vi "温度补偿.vi"() -> ()   [LabVIEW 2016, in "斯坦道CODMn.lvlib"]
uses:
  <vilib>/Analysis/6fits.llb/Curve Fitting Criteria.ctl
  <vilib>/Plasmionique/MB Master/MB Master.lvlib
  <vilib>/Analysis/NI_AALPro.lvlib
panel:
  in  "读取":bool
  in  "写入":bool
  in  "关闭":bool
  in  "曲线模型":T1 {"二次方程"."x^2" format="%#.6g"; "二次方程"."K" format="%#.6g"; "二次方程"."B" format="%#.6g"; "r^2" format="%.7f"; "测量吸光度5" format="%#.6f"; "测量吸光度4" format="%#.6f"; "测量吸光度3" format="%#.6f"; "测量吸光度2" format="%#.6f"; "测量吸光度1" format="%#.6f"}
  # "温度"
  # "滴定数"
  # "温度一"
  # "温度二"
  # "温度三"
  # "温度四"
  # "温度五"
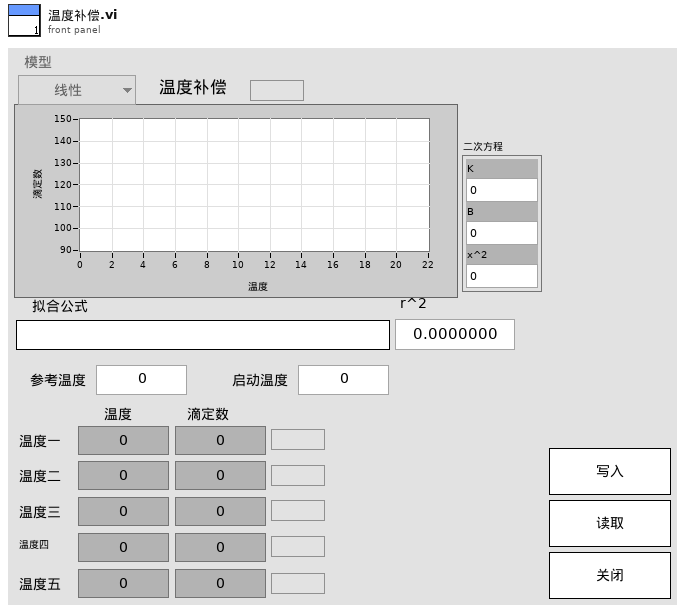
[diagram p1: front panel]
types:
  T1 = cluster{"标液浓度1":dbl, "测量吸光度1":dbl, "样品1启用":bool, "标液浓度2":dbl, "测量吸光度2":dbl, "样品2启用":bool, "标液浓度3":dbl, "测量吸光度3":dbl, "样品3启用":bool, "标液浓度4":dbl, "测量吸光度4":dbl, "样品4启用":bool, "标液浓度5":dbl, "测量吸光度5":dbl, "样品5启用":bool, "模型":enum32{"线性", "多项式", "折线"}, "XY图":cluster{"X Values":dbl[], "Y Values":dbl[]}[], "拟合公式":string, "r^2":dbl, "二次方程":cluster{"K":dbl, "B":dbl, "x^2":dbl}, "参考温度":dbl, "温度补偿":bool, "启动温度":dbl}
  T2 = typedef "NI_AALPro.lvlib/Curve Fitting Criteria.ctl" = u16
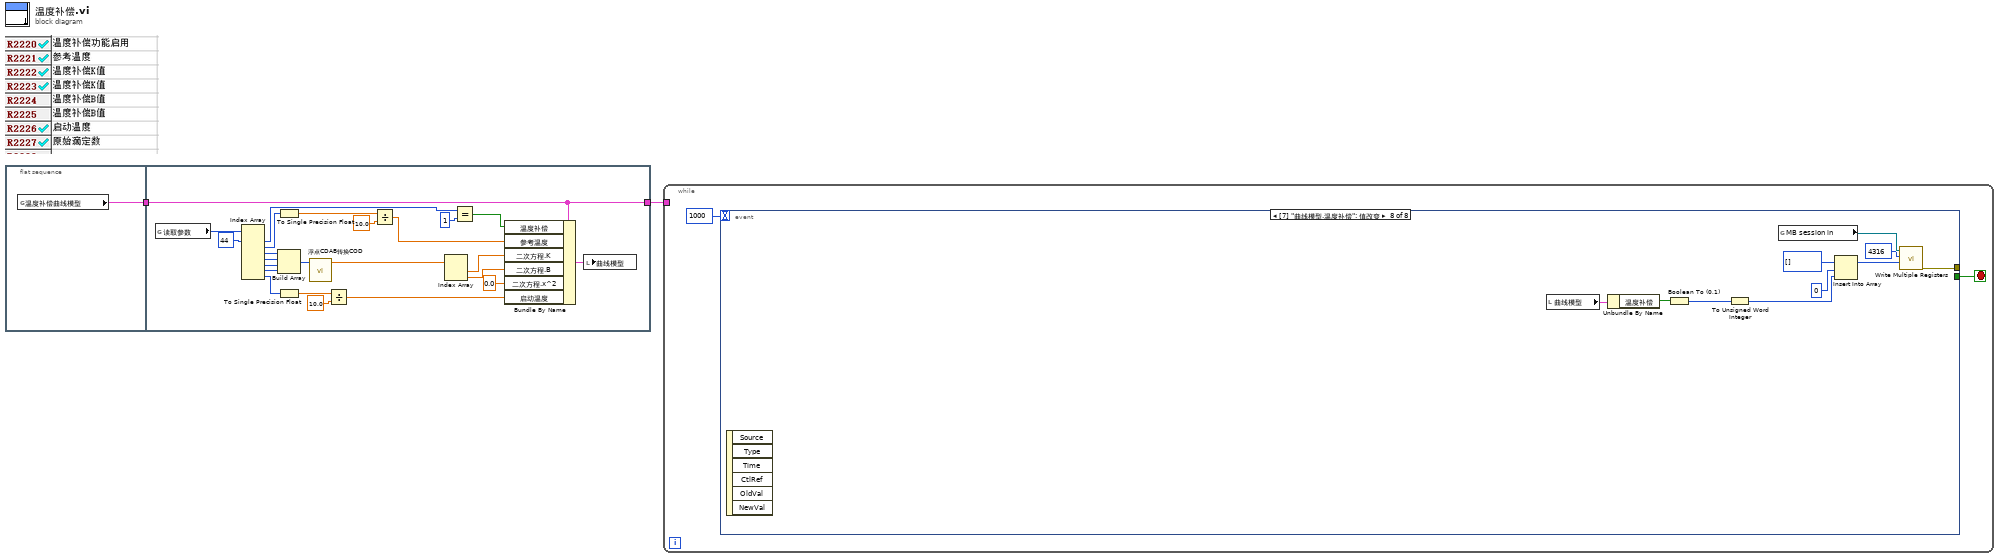
[diagram p0: block diagram]
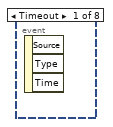
[diagram p2: hidden frame]
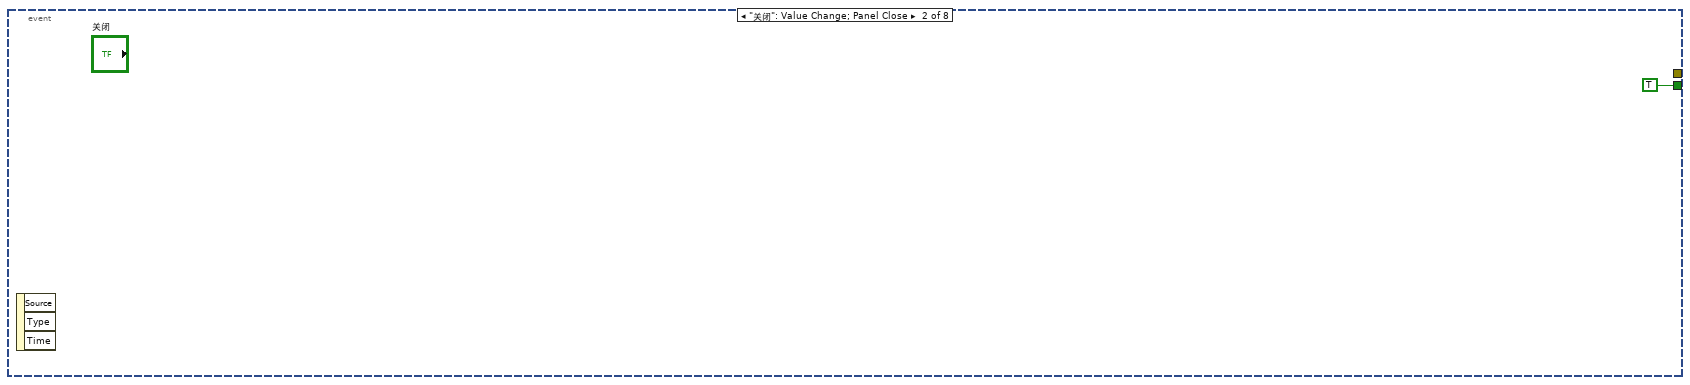
[diagram p3: hidden frame]
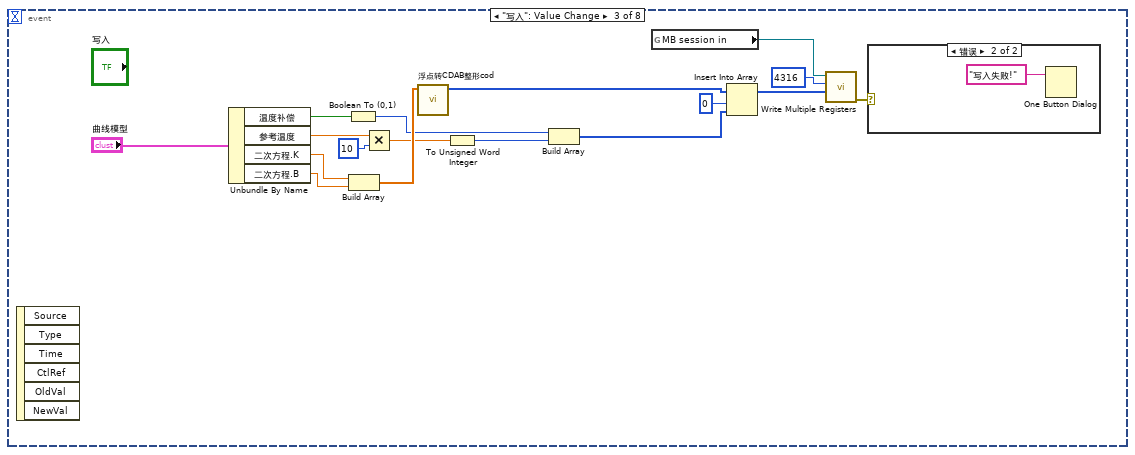
[diagram p4: hidden frame]
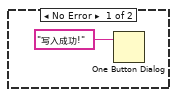
[diagram p5: hidden frame]
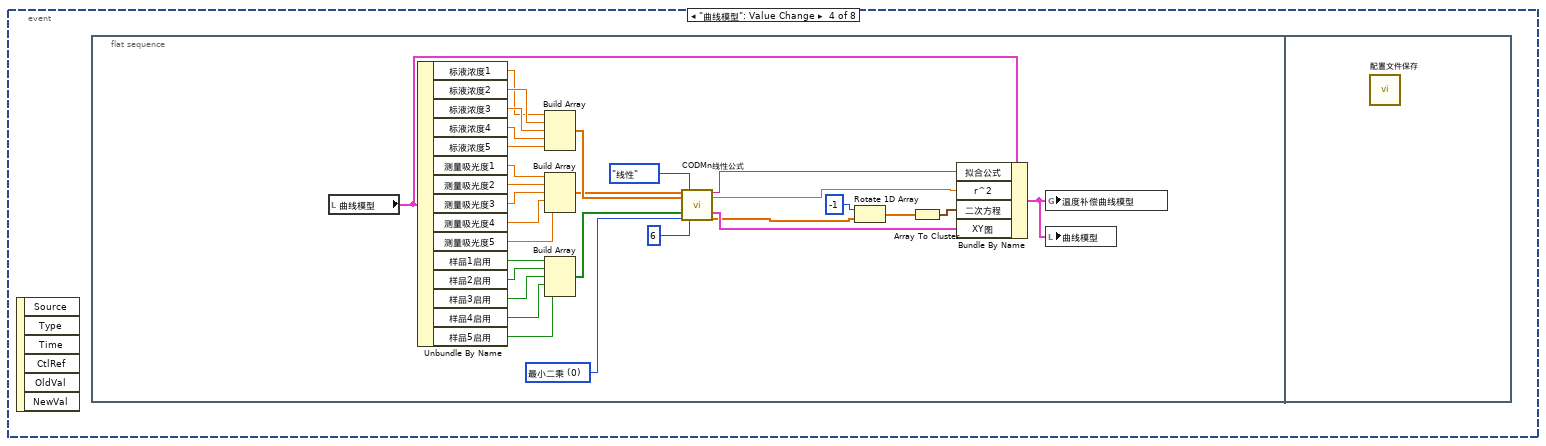
[diagram p6: hidden frame]
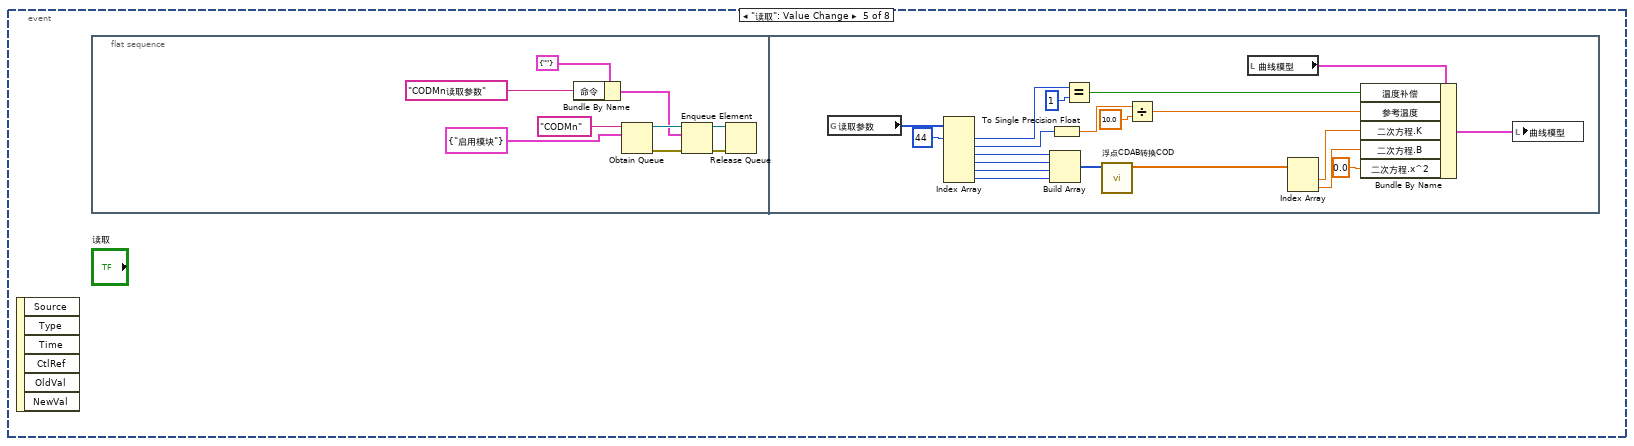
[diagram p7: hidden frame]
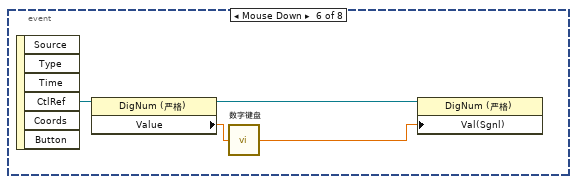
[diagram p8: hidden frame]
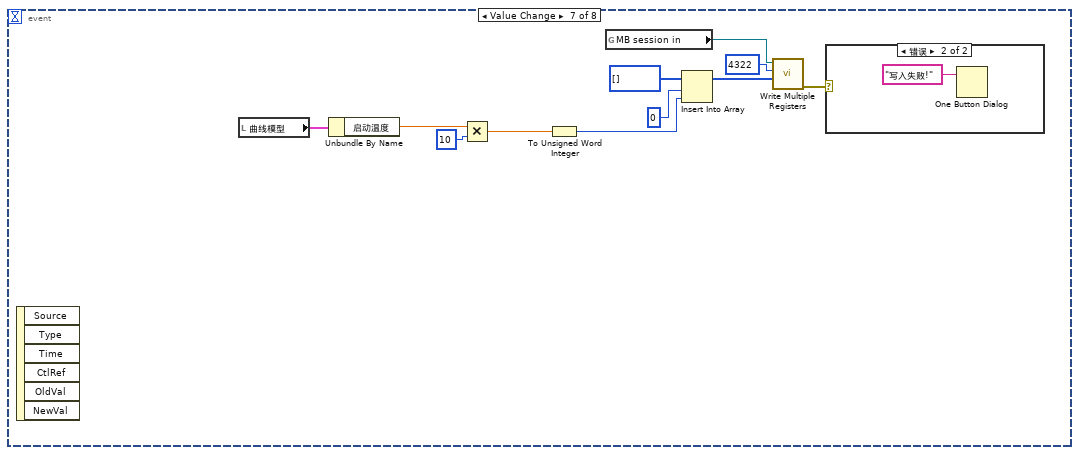
[diagram p9: hidden frame]
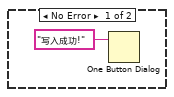
[diagram p10: hidden frame]
diagram:
  n1 = flat-sequence {
    tunnel: [w3] -> w1
    tunnel: [w25] -> w2
    tunnel: w1 -> [w25]
    frame #0 {
      n2 = global read "CODMn断电保存全局变量.vi" "温度补偿曲线模型"() -> (w3:T1)
    }
    frame #1 {
      n3 = global read "COD内部交互全局.vi" "读取参数"() -> (w27:u16[])
      n4 = Index Array(array=w27, index #1=44 ("索引")) -> (element #1=w12:u16, element #2=w9:u16, element #3=w22:u16, element #4=w21:u16, element #5=w20:u16, element #6=w19:u16, element #7=w5:u16)  [unwired: 6 in]
      n5 = To Single Precision Float(number=w9) -> (single precision float=w8:sgl)
      n6 = Build Array(w22, w21, w20, w19) -> (w18:u16[])
      n7 = To Single Precision Float(number=w5) -> (single precision float=w7:sgl)
      n8 = call "浮点CDAB转换COD.vi"("数组"=w18) -> ("数组 2"=w17:sgl[])  [unwired: 10 in]
      n9 = Divide(x=w7, y=sgl 10.0) -> (x/y=w4:sgl)
      n10 = Divide(x=w8, y=sgl 10.0) -> (x/y=w23:sgl)
      n11 = Index Array(array=w17) -> (element #1=w16:sgl, element #2=w15:sgl)  [unwired: 2 in]
      n12 = Equal?(x=w12, y=u16 1) -> (x = y?=w10:bool)
      n13 = Bundle By Name(cluster=w25, "温度补偿"=w10, "参考温度"=w23, "二次方程.K"=w16, "二次方程.B"=w15, "二次方程.x^2"=0.0, "启动温度"=w4) -> (w24:T1)
      n14 = local write "曲线模型"(w24) -> ()
    }
  }
  n15 = while {
    tunnel: w2 -> [_]
    stop <- w29 stop-if-true
    n16 = event shown="[7] \"曲线模型.温度补偿\": 值改变" {
      selector: _ -> [_ _ _ _ _ _ _ _]
      dyn-events: _ -> [_ _ _ _ _ _ _ _]
      timeout: 1000 -> [_ _ _ _ _ _ _ _]
      tunnel: [_ TRUE _ _ _ _ _ _] -> w29
      tunnel: [_ _ _ _ _ _ _ w126] -> _
      event Timeout {
        n17 = event-data() -> ()  [unwired: 1 in, 3 out]
      }
      event "关闭": Value Change; Panel Close {
        n18 = event-data() -> ()  [unwired: 1 in, 3 out]
      }
      event "写入": Value Change {
        n19 = event-data() -> ()  [unwired: 1 in, 6 out]
        n20 = Unbundle By Name("曲线模型") -> ("温度补偿"=w34:bool, "参考温度"=w40:dbl, "二次方程.K"=w44:dbl, "二次方程.B"=w43:dbl)
        n21 = Boolean To (0,1)(Boolean=w34) -> (0, 1=w33:i16)
        n22 = Build Array(w44, w43) -> (w42:dbl[])
        n23 = Multiply(x=w40, y=u16 10 ("新元素/子数组")) -> (x*y=w38:dbl)
        n24 = call "浮点转CDAB整形cod.vi"("浮点数"=w42) -> ("CDAB整形输出"=w31:u16[])  [unwired: 10 in]
        n25 = To Unsigned Word Integer(number=w38) -> (unsigned 16bit integer=w35:u16)
        n26 = Build Array(w33, w35) -> (w32:u16[])
        n27 = global read "COD浓度全局变量.vi" "MB session in"() -> (w46:refnum<class "MB_Master.lvclass">)
        n28 = Insert Into Array(array=w31, index=0 ("索引"), new element=w32) -> (w37:u16[])
        n29 = call <vilib>:"Write Multiple Registers.vi"("values"=w37, "starting address"=u16 4316, "MB session in"=w46) -> ("error out"=w36:errorcluster)  [unwired: 7 in, 1 out]
        n30 = case shown="错误" w36 {
          frame No Error {
            n31 = One Button Dialog(message="写入成功!" ("消息")) -> ()  [unwired: 1 in, 1 out]
          }
          frame Error {
            n32 = One Button Dialog(message="写入失败!" ("消息")) -> ()  [unwired: 1 in, 1 out]
          }
        }
      }
      event "曲线模型": Value Change {
        n33 = event-data() -> ()  [unwired: 1 in, 6 out]
        n34 = flat-sequence {
          frame #0 {
            w51 = T2 0 items=["最小二乘", "最小绝对残差", "Bisquare"] ("method")
            n35 = local read "曲线模型"() -> (w72:T1)
            n36 = Unbundle By Name(w72) -> ("标液浓度1"=w54:dbl, "标液浓度2"=w55:dbl, "标液浓度3"=w56:dbl, "标液浓度4"=w57:dbl, "标液浓度5"=w58:dbl, "测量吸光度1"=w59:dbl, "测量吸光度2"=w60:dbl, "测量吸光度3"=w61:dbl, "测量吸光度4"=w62:dbl, "测量吸光度5"=w63:dbl, "样品1启用"=w64:bool, "样品2启用"=w65:bool, "样品3启用"=w66:bool, "样品4启用"=w67:bool, "样品5启用"=w68:bool)
            n37 = Build Array(w54, w55, w56, w57, w58) -> (w71:dbl[])
            n38 = Build Array(w59, w60, w61, w62, w63) -> (w70:dbl[])
            n39 = Build Array(w64, w65, w66, w67, w68) -> (w69:bool[])
            n40 = call "CODMn线性公式.vi"("标液浓度"=w70, "滴定数"=w71, "启用"=w69, "method"=w51, "模型"=enum32{"线性", "多项式", "折线"}."线性", "精度"=6) -> ("拟合方程"=w73:string, "r^2"=w74:dbl, "XY图"=w79:cluster{"X Values":dbl[], "Y Values":dbl[]}[], "Polynomial Coefficients"=w78:dbl[])  [unwired: 7 in, 3 out]
            n41 = Rotate 1D Array(1:w78, 2:-1 ("n")) -> (0:w75:dbl[])
            n42 = Array To Cluster(array=w75) -> (cluster=w77:cluster{"[0]":dbl, "[1]":dbl, "[2]":dbl})
            n43 = Bundle By Name(cluster=w72, "拟合公式"=w73, "r^2"=w74, "二次方程"=w77, "XY图"=w79) -> (w50:T1)
            n44 = global write "CODMn断电保存全局变量.vi" "温度补偿曲线模型"(w50) -> ()
            n45 = local write "曲线模型"(w50) -> ()
          }
          frame #1 {
            n46 = call "配置文件保存.vi"() -> ()  [unwired: 12 in]
          }
        }
      }
      event "读取": Value Change {
        n47 = event-data() -> ()  [unwired: 1 in, 6 out]
        n48 = flat-sequence {
          frame #0 {
            n49 = Bundle By Name(cluster=cluster{"命令":string} {"命令"=""} ("元素"), "命令"="CODMn读取参数" ("名称（未命名）")) -> (w82:cluster{"命令":string})
            n50 = Obtain Queue(name (unnamed)="CODMn", element data type=cluster{"命令":string} {"命令"="启用模块"} ("元素")) -> (queue out=w87:refnum<queue>, error out=w88:errorcluster)  [unwired: 3 in, 1 out]
            n51 = Enqueue Element(queue=w87, element=w82, error in (no error)=w88) -> (queue out=w85:refnum<queue>, error out=w86:errorcluster)  [unwired: 1 in, 1 out]
            n52 = Release Queue(queue=w85, error in (no error)=w86) -> ()  [unwired: 1 in, 3 out]
          }
          frame #1 {
            n53 = global read "COD内部交互全局.vi" "读取参数"() -> (w92:u16[])
            n54 = Index Array(array=w92, index #1=44 ("索引")) -> (element #1=w106:u16, element #2=w90:u16, element #3=w96:u16, element #4=w97:u16, element #5=w98:u16, element #6=w99:u16)  [unwired: 5 in]
            n55 = Build Array(w96, w97, w98, w99) -> (w100:u16[])
            n56 = To Single Precision Float(number=w90) -> (single precision float=w89:sgl)
            n57 = Equal?(x=w106, y=u16 1) -> (x = y?=w108:bool)
            n58 = call "浮点CDAB转换COD.vi"("数组"=w100) -> ("数组 2"=w101:sgl[])  [unwired: 10 in]
            n59 = Divide(x=w89, y=sgl 10.0) -> (x/y=w95:sgl)
            n60 = local read "曲线模型"() -> (w91:T1)
            n61 = Index Array(array=w101) -> (element #1=w102:sgl, element #2=w103:sgl)  [unwired: 2 in]
            n62 = Bundle By Name(cluster=w91, "温度补偿"=w108, "参考温度"=w95, "二次方程.K"=w102, "二次方程.B"=w103, "二次方程.x^2"=0.0) -> (w94:T1)
            n63 = local write "曲线模型"(w94) -> ()
          }
        }
      }
      event "曲线模型.标液浓度1", "曲线模型.测量吸光度1", "曲线模型.标液浓度2", "曲线模型.测量吸光度2", "曲线模型.标液浓度3", "曲线模型.测量吸光度3", "曲线模型.标液浓度4", "曲线模型.测量吸光度4", "曲线模型.标液浓度5", "曲线模型.测量吸光度5", "曲线模型.参考温度", "曲线模型.启动温度": Mouse Down {
        n64 = event-data() -> ("CtlRef"=w112:refnum<vi>)  [unwired: 1 in, 5 out]
        n65 = property class="DigNum (严格)"(reference=w112) -> (reference out=w110:refnum<vi>, "Value"=w111:dbl)  [unwired: 1 in, 1 out]
        n66 = call "数字键盘.vi"("OldNumber"=w111) -> ("NewNumber"=w109:sgl)
        n67 = property class="DigNum (严格)"(reference=w110, "Val(Sgnl)"=w109) -> ()  [unwired: 1 in, 2 out]
      }
      event "曲线模型.启动温度": Value Change {
        n68 = event-data() -> ()  [unwired: 1 in, 6 out]
        n69 = local read "曲线模型"() -> (w123:T1)
        n70 = Unbundle By Name(w123) -> ("启动温度"=w115:dbl)
        n71 = Multiply(x=w115, y=u16 10 ("新元素/子数组")) -> (x*y=w116:dbl)
        n72 = To Unsigned Word Integer(number=w116) -> (unsigned 16bit integer=w114:u16)
        n73 = global read "COD浓度全局变量.vi" "MB session in"() -> (w122:refnum<class "MB_Master.lvclass">)
        n74 = Insert Into Array(array=u16[] [] ("CDAB整形输出"), index=0 ("索引"), new element=w114) -> (w119:u16[])
        n75 = call <vilib>:"Write Multiple Registers.vi"("values"=w119, "starting address"=u16 4322, "MB session in"=w122) -> ("error out"=w113:errorcluster)  [unwired: 7 in, 1 out]
        n76 = case shown="错误" w113 {
          frame No Error {
            n77 = One Button Dialog(message="写入成功!" ("消息")) -> ()  [unwired: 1 in, 1 out]
          }
          frame Error {
            n78 = One Button Dialog(message="写入失败!" ("消息")) -> ()  [unwired: 1 in, 1 out]
          }
        }
      }
      event "曲线模型.温度补偿": Value Change {
        n79 = event-data() -> ()  [unwired: 1 in, 6 out]
        n80 = local read "曲线模型"() -> (w135:T1)
        n81 = Unbundle By Name(w135) -> ("温度补偿"=w128:bool)
        n82 = Boolean To (0,1)(Boolean=w128) -> (0, 1=w127:i16)
        n83 = To Unsigned Word Integer(number=w127) -> (unsigned 16bit integer=w130:u16)
        n84 = global read "COD浓度全局变量.vi" "MB session in"() -> (w134:refnum<class "MB_Master.lvclass">)
        n85 = Insert Into Array(array=u16[] [] ("CDAB整形输出"), index=0 ("索引"), new element=w130) -> (w132:u16[])
        n86 = call <vilib>:"Write Multiple Registers.vi"("values"=w132, "starting address"=u16 4316, "MB session in"=w134) -> ("error out"=w126:errorcluster)  [unwired: 7 in, 1 out]
      }
    }
  }
